vi "Access insert values.vi"(5 "是否创建唯一键":bool, 6 "Password":string, 7 "data":variant[](array[variant]), 8 "error in (no error)":errorcluster, 9 "columns外部输入":T1, 10 "database":string="database1.mdb", 11 "table":string) -> (0 "error out":errorcluster)   [LabVIEW 2016, in "Access Lib.lvlib"]
uses:
  Access Lib.lvlib
  <vilib>/addons/database/Auxilliary.llb/DB Tools Transaction.ctl
  <vilib>/addons/database/Auxilliary.llb/DB Tools Isolation Level.ctl
  <vilib>/addons/database/Auxilliary.llb/DB Tools Column Info.ctl
  <vilib>/addons/database/Auxilliary.llb/DB Tools DataTypes.ctl
  <vilib>/addons/database/Auxilliary.llb/DB Tools Parameter Info.ctl
  <vilib>/addons/database/Auxilliary.llb/DB Tools Parameter Dir.ctl
  <vilib>/addons/database/Connection.llb/DB Tools Open Connec (String).vi
  <vilib>/addons/database/Connection.llb/Conn Transaction.vi
  <vilib>/addons/database/Connection.llb/Conn Execute.vi
  <vilib>/addons/database/Recordset.llb/Rec Destroy - Connection.vi
  <vilib>/addons/database/Command.llb/Cmd Set Parameter Value (C).vi
  <vilib>/addons/database/Command.llb/Cmd Execute.vi
  <vilib>/addons/database/Recordset.llb/Rec Destroy - Command.vi
  <vilib>/addons/database/Command.llb/Cmd Delete.vi
  <vilib>/addons/database/NI_Database_API.lvlib
  <vilib>/Utility/VariantDataType/VariantType.lvlib
panel:
  out "SN":string
  out "布尔":bool
  out "曲线截距":sgl
  out "曲线斜率":sgl
  out "二次多项式系数":sgl
  out "X":sgl
  out "检测值":sgl
  out "测试模式":enum16{"水样测试", "零点核查", "跨度核查"}(ring)
  out "当前数据时间":timestamp
  out "当前测量模式":string
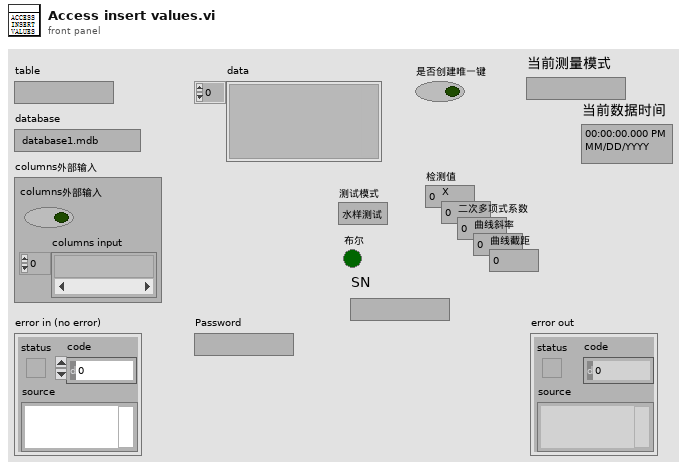
[diagram p1: front panel]
types:
  T1 = cluster{"columns外部输入":bool, "columns input":string[]}
  T2 = typedef "NI_Database_API.lvlib/DB Tools Isolation Level.ctl" = enum16{"chaos", "read uncommitted", "read committed", "repeatable read", "serializable"}
  T3 = typedef "NI_Database_API.lvlib/DB Tools Transaction.ctl" = enum16{"begin", "commit", "rollback"}
  T4 = typedef "NI_Database_API.lvlib/DB Tools Column Info.ctl" = cluster{"column name":string, "data type":T5, "size":i32, "allow null?":bool}
  T5 = typedef "NI_Database_API.lvlib/DB Tools DataTypes.ctl" = enum16{"String", "Long (I32)", "Single (SGL)", "Double (DBL)", "Date/Time", "Binary"}
  T6 = typedef "VariantType.lvlib/Type.ctl" = enum8{"Invalid Type", "Void", "I8", "I16", "I32", "I64", "U8", "U16", "U32", "U64", "Single Float", "Double Float", "Extended Float", "Single Complex", "Double Complex", "Extended Complex", "Enum U8", "Enum U16", "Enum U32", "Enum U64", "Single Float With Unit", "Double Float With Unit", "Extended Float With Unit", "Single Complex with Unit", "Double Complex with Unit", "Extended Complex with Unit", "Boolean", "String", "Path", "Picture", "Tag", "Array", "Cluster", "Variant", "LV Variant", "Waveform", "Timestamp", "Digital Waveform", "Digital Data", "ExpressData", "Refnum", "External Data", "VI", "Poly VI", "LabVIEW Class Instance", "Fixed Point"}
  T7 = typedef "NI_Database_API.lvlib/Conn ObjectReference.ctl" = refnum<k1>
  T8 = typedef "NI_Database_API.lvlib/DB Tools Parameter Info.ctl" = cluster{"parameter name":string, "type":T5, "direction":T9, "value":variant}
  T9 = typedef "NI_Database_API.lvlib/DB Tools Parameter Dir.ctl" = enum32{"Input", "Output", "Input/Output", "Return Value"}
  T10 = typedef "NI_Database_API.lvlib/Rec ObjectReference.ctl" = refnum<k1>
  T11 = typedef "LVDateTimeRec.ctl" = cluster{"秒数的小数部分":dbl, "秒":i32, "分":i32, "时":i32, "日":i32, "月":i32, "年":i32, "天数（周）":i32, "天数（年）":i32, "DST":i32}
  T12 = typedef "NI_Database_API.lvlib/Cmd ObjectReference.ctl" = refnum<k1>
  T13 = typedef "NI_Database_API.lvlib/Cmd-Rec Object Reference.ctl" = refnum<k1>
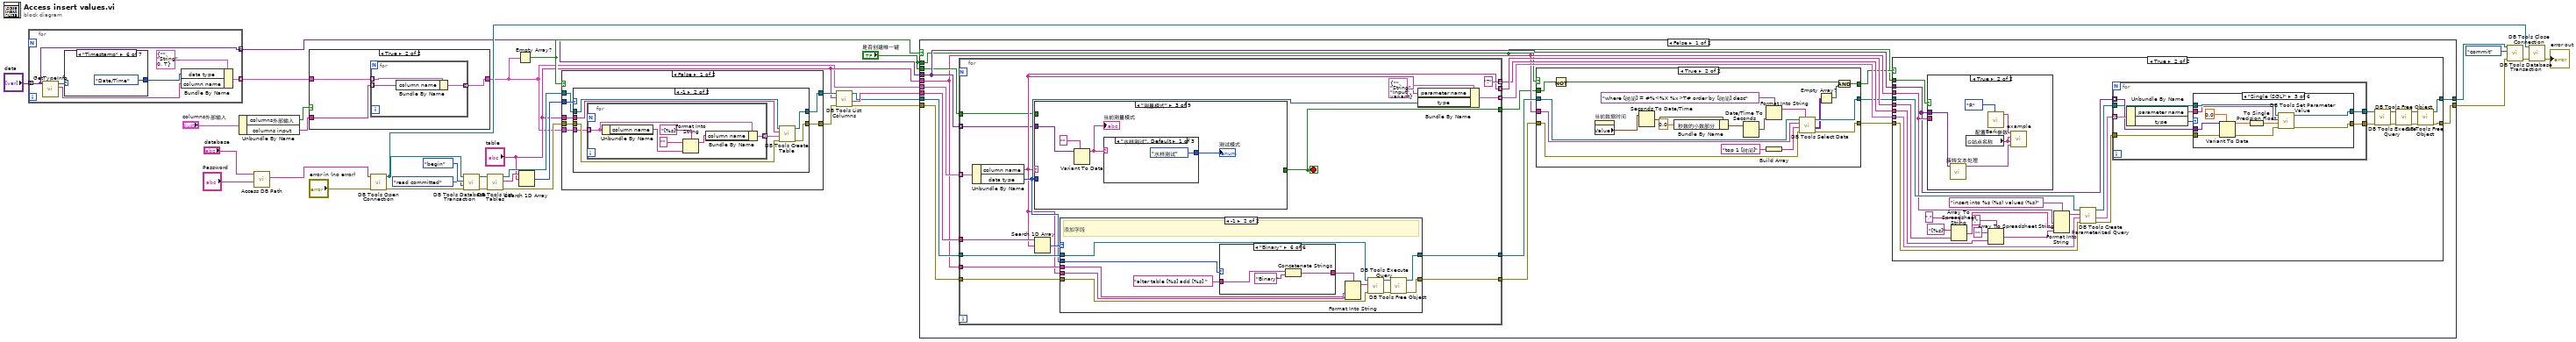
[diagram p0: block diagram]
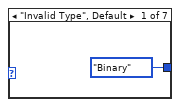
[diagram p3: hidden frame]
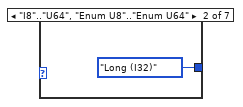
[diagram p4: hidden frame]
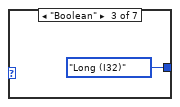
[diagram p5: hidden frame]
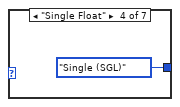
[diagram p6: hidden frame]
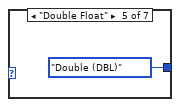
[diagram p7: hidden frame]
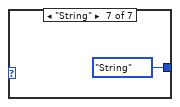
[diagram p8: hidden frame]
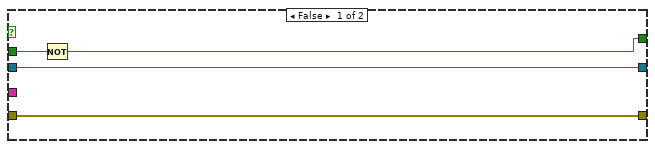
[diagram p11: hidden frame]
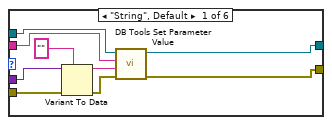
[diagram p14: hidden frame]
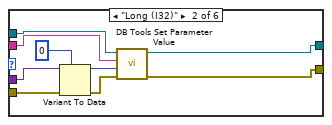
[diagram p15: hidden frame]
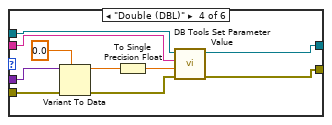
[diagram p16: hidden frame]
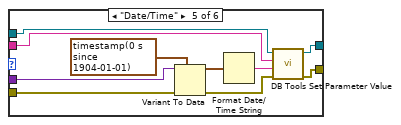
[diagram p17: hidden frame]
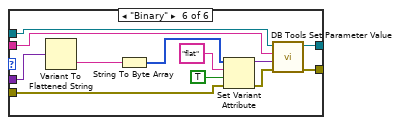
[diagram p18: hidden frame]
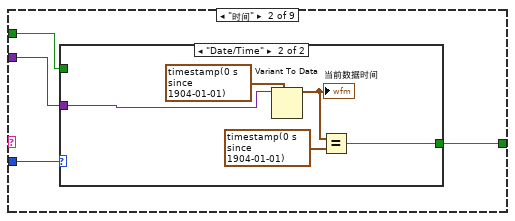
[diagram p20: hidden frame]
diagram:
  n1 = for {
    tunnel: [w35] -> w12 mode=indexing
    tunnel: [w37] -> w9 mode=indexing
    tunnel: "data" -> [w35] mode=indexing
    n2 = call <vilib>:"GetTypeInfo.vi"("Variant"=w35) -> ("Name"=w36:string, "Type Enum"=w39:T6)  [unwired: 6 in, 3 out]
    n3 = case shown="\"Timestamp\"" w39 {
      tunnel: [DB_Tools_DataTypes."Binary" ("data type") DB_Tools_DataTypes."Long (I32)" ("data type") DB_Tools_DataTypes."Long (I32)" ("data type") DB_Tools_DataTypes."Single (SGL)" ("data type") DB_Tools_DataTypes."Double (DBL)" ("data type") DB_Tools_DataTypes."Date/Time" ("data type") DB_Tools_DataTypes."String" ("data type")] -> w38
      frame "Invalid Type", Default {
      }
      frame "I8".."U64", "Enum U8".."Enum U64" {
      }
      frame "Boolean" {
      }
      frame "Single Float" {
      }
      frame "Double Float" {
      }
      frame "Timestamp" {
      }
      frame "String" {
      }
    }
    n4 = Bundle By Name(cluster=T4 {"column name"="", "data type"=enum."String", "size"=0, "allow null?"=TRUE} ("column information"), "data type"=w38, "column name"=w36) -> (w37:T4)
  }
  n5 = Unbundle By Name("columns外部输入") -> ("columns外部输入"=w7:bool, "columns input"=w8:string[])
  n6 = call "Access DB Path.vi"("Password"="Password", "database"="database") -> ("Connection information"=w5:string)  [unwired: 8 in, 1 out]
  n7 = case shown="True" w7 {
    tunnel: w9 -> [w48 w51]
    tunnel: [w48 w50] -> w6
    tunnel: w8 -> [_ w49]
    frame False {
    }
    frame True {
      n8 = for {
        tunnel: w51 -> [w54] mode=indexing
        tunnel: [w53] -> w50 mode=indexing
        tunnel: w49 -> [w52] mode=indexing
        n9 = Bundle By Name(cluster=w54, "column name"=w52) -> (w53:T4)
      }
    }
  }
  n10 = call-poly <vilib>:"DB Tools Open Connection.vi"("error in (no error)"="error in (no error)", "connection information"=w5) -> ("error out"=w19:errorcluster, "connection reference"=w16:T7)  [unwired: 6 in]
  n11 = call-poly <vilib>:"DB Tools Database Transaction.vi"("error in (no error)"=w19, "isolation level (chaos)"=DB_Tools_Isolation_Level."read committed", "operation (begin)"=DB_Tools_Transaction."begin", "connection reference"=w16) -> ("error out"=w18:errorcluster, "connection reference out"=w20:T7)  [unwired: 2 in]
  n12 = call <vilib>:"DB Tools List Tables.vi"("error in (no error)"=w18, "connection reference"=w20) -> ("error out"=w27:errorcluster, "tables"=w29:string[], "connection reference out"=w17:T7)  [unwired: 3 in]
  n13 = Empty Array?(array=w6) -> (empty?=w14:bool)
  n14 = Search 1D Array(1D array=w29, element="table") -> (index of element=w28:i32)  [unwired: 1 in]
  n15 = case shown="False" w14 {
    tunnel: w28 -> [w61 _]
    tunnel: w27 -> [w60 w77]
    tunnel: [w59 w78] -> w25
    tunnel: [w58 w77] -> w24
    tunnel: w17 -> [w57 w78]
    tunnel: "table" -> [w56 _]
    tunnel: w6 -> [w55 _]
    frame False {
      n16 = case shown="-1" w61 {
        tunnel: w57 -> [w63 w70]
        tunnel: w60 -> [w62 w69]
        tunnel: w56 -> [_ w68]
        tunnel: w55 -> [_ w65]
        tunnel: [w63 w67] -> w59
        tunnel: [w62 w66] -> w58
        frame 0, Default {
        }
        frame -1 {
          n17 = for {
            tunnel: w65 -> [w72] mode=indexing
            tunnel: [w71] -> w64 mode=indexing
            n18 = Unbundle By Name(w72) -> ("column name"=w76:string)
            n19 = Format Into String(format string="[%s]" ("格式字符串"), initial string="" ("初始字符串"), w76) -> (resulting string=w73:string)  [unwired: 1 in, 1 out]
            n20 = Bundle By Name(cluster=w72, "column name"=w73) -> (w71:T4)
          }
          n21 = call <vilib>:"DB Tools Create Table.vi"("error in (no error)"=w69, "column information"=w64, "table"=w68, "connection reference"=w70) -> ("error out"=w66:errorcluster, "connection reference out"=w67:T7)  [unwired: 4 in]
        }
      }
    }
    frame True {
    }
  }
  n22 = call <vilib>:"DB Tools List Columns.vi"("error in (no error)"=w24, "table"="table", "connection reference"=w25) -> ("error out"=w3:errorcluster, "columns"=w26:string[], "connection reference out"=w4:T7)  [unwired: 1 in, 1 out]
  n23 = case shown="False" w14 {
    tunnel: w26 -> [w97 _]
    tunnel: w3 -> [w96 w306]
    tunnel: [w92 w307] -> w22
    tunnel: [w91 w306] -> w21
    tunnel: w12 -> [w88 _]
    tunnel: w4 -> [w90 w307]
    tunnel: "table" -> [w82 _]
    tunnel: w6 -> [w89 _]
    tunnel: "是否创建唯一键" -> [w87 _]
    tunnel: "是否创建唯一键" -> [w79 _]
    frame False {
      n24 = for {
        tunnel: w90 -> [w236]
        tunnel: w97 -> [w238]
        tunnel: w96 -> [w235]
        tunnel: [w234] -> w84
        tunnel: w82 -> [w233]
        tunnel: w89 -> [w232] mode=indexing
        tunnel: [w230] -> w95 mode=indexing
        tunnel: [w226] -> w94 mode=indexing
        tunnel: ["?"] -> w93 mode=indexing
        tunnel: [w228] -> w86
        tunnel: w88 -> [w225] mode=indexing
        tunnel: [w224] -> w81
        tunnel: w87 -> [w223]
        stop <- w224 stop-if-true
        n25 = Unbundle By Name(w232) -> ("column name"=w226:string, "data type"=w227:T5)
        n26 = case shown="\"测量模式\"" w226 {
          tunnel: w227 -> [_ w242 _ _ _ _ _ _ _]
          tunnel: w225 -> [_ w241 w251 w257 w260 w263 w266 w269 w272]
          tunnel: [_ w240 _ _ _ _ _ _ _] -> w224
          tunnel: w223 -> [_ w239 _ _ _ _ _ _ _]
          frame "假", Default {
          }
          frame "时间" {
            n27 = case shown="\"Date/Time\"" w242 {
              tunnel: w241 -> [_ w247]
              tunnel: [_ w243] -> w240
              tunnel: w239 -> [_ _]
              frame "String", Default {
              }
              frame "Date/Time" {
                n28 = Variant To Data(type=timestamp(0 s since 1904-01-01) ("时间标识"), Variant=w247) -> (data=w245:timestamp)  [unwired: 1 in, 1 out]
                "当前数据时间" <- w245
                n29 = Equal?(x=w245, y=timestamp(0 s since 1904-01-01) ("时间标识")) -> (x = y?=w243:bool)
              }
            }
          }
          frame "测量模式" {
            n30 = Variant To Data(type="", Variant=w251) -> (data=w249:string)  [unwired: 1 in, 1 out]
            "当前测量模式" <- w249
            n31 = case shown="\"水样测试\", Default" w249 {
              tunnel: [enum16{"水样测试", "零点核查", "跨度核查"}."水样测试" ("测试模式") enum16{"水样测试", "零点核查", "跨度核查"}."零点核查" ("测试模式") enum16{"水样测试", "零点核查", "跨度核查"}."跨度核查" ("测试模式")] -> w248
              frame "水样测试", Default {
              }
              frame "零点核查" {
              }
              frame "跨度核查" {
              }
            }
            "测试模式" <- w248
          }
          frame "检测值" {
            n32 = Variant To Data(type=sgl 0.0, Variant=w257) -> (data=→"检测值":sgl)  [unwired: 1 in, 1 out]
            "布尔" <- TRUE ("布尔")
          }
          frame "X0" {
            n33 = Variant To Data(type=sgl 0.0, Variant=w260) -> (data=→"X":sgl)  [unwired: 1 in, 1 out]
          }
          frame "二次多项式系数" {
            n34 = Variant To Data(type=sgl 0.0, Variant=w263) -> (data=→"二次多项式系数":sgl)  [unwired: 1 in, 1 out]
          }
          frame "曲线斜率" {
            n35 = Variant To Data(type=sgl 0.0, Variant=w266) -> (data=→"曲线斜率":sgl)  [unwired: 1 in, 1 out]
          }
          frame "曲线截距" {
            n36 = Variant To Data(type=sgl 0.0, Variant=w269) -> (data=→"曲线截距":sgl)  [unwired: 1 in, 1 out]
          }
          frame "SN" {
            n37 = Variant To Data(type="", Variant=w272) -> (data=→"SN":string)  [unwired: 1 in, 1 out]
          }
        }
        n38 = Search 1D Array(1D array=w238, element=w226) -> (index of element=w237:i32)  [unwired: 1 in]
        n39 = case shown="-1" w237 {
          tunnel: [w275 w284] -> w234
          tunnel: w236 -> [w274 w283]
          tunnel: w226 -> [_ w282]
          tunnel: w235 -> [w275 w281]
          tunnel: w233 -> [_ w280]
          tunnel: w227 -> [_ w278]
          tunnel: [w274 w276] -> w228
          frame 0, Default {
          }
          frame -1 {
            # "添加字段"
            n40 = case shown="\"Binary\"" w278 {
              tunnel: "alter table [%s] add [%s] " -> [w290 w293 w296 w299 w302 w305]
              tunnel: [w289 w292 w295 w298 w301 w304] -> w277
              frame "String", Default {
                n41 = Concatenate Strings(w290, "String" ("字符串")) -> (w289:string)
              }
              frame "Long (I32)" {
                n42 = Concatenate Strings(w293, "Long" ("字符串")) -> (w292:string)
              }
              frame "Single (SGL)" {
                n43 = Concatenate Strings(w296, "Single" ("字符串")) -> (w295:string)
              }
              frame "Double (DBL)" {
                n44 = Concatenate Strings(w299, "Double" ("字符串")) -> (w298:string)
              }
              frame "Date/Time" {
                n45 = Concatenate Strings(w302, "TimeStamp" ("字符串")) -> (w301:string)
              }
              frame "Binary" {
                n46 = Concatenate Strings(w305, "Binary" ("字符串")) -> (w304:string)
              }
            }
            n47 = Format Into String(format string=w277, w280, w282) -> (resulting string=w285:string)  [unwired: 2 in, 1 out]
            n48 = call-poly <vilib>:"DB Tools Execute Query.vi"("error in (no error)"=w281, "SQL query"=w285, "connection reference"=w283) -> ("error out"=w286:errorcluster, "recordset reference"=w287:T10)  [unwired: 5 in]
            n49 = call-poly <vilib>:"DB Tools Free Object.vi"("error in (no error)"=w286, "recordset reference"=w287) -> ("error out"=w284:errorcluster, "connection reference"=w276:T7)  [unwired: 8 in]
          }
        }
        n50 = Bundle By Name(cluster=T8 {"parameter name"="", "type"=enum."String", "direction"=enum."Input", "value"=variant} ("parameter information"), "parameter name"=w226, "type"=w227) -> (w230:T8)
      }
      n51 = case shown="True" w79 {
        tunnel: w86 -> [w101 w118]
        tunnel: [w101 w117] -> w85
        tunnel: w84 -> [w100 w116]
        tunnel: [w100 w115] -> w83
        tunnel: w82 -> [_ w114]
        tunnel: w81 -> [w99 w103]
        tunnel: [w98 w105] -> w80
        frame False {
          n52 = Not(x=w99) -> (.not. x?=w98:bool)
        }
        frame True {
          n53 = Not(x=w103) -> (.not. x?=w102:bool)
          n54 = property on="当前数据时间" class="AbsTime (strict)"() -> ("Value"=w111:timestamp)  [unwired: 2 in, 2 out]
          n55 = Seconds To Date/Time(time stamp (now)=w111) -> (date time rec=w110:T11)  [unwired: 1 in]
          n56 = Bundle By Name(cluster=w110, "秒数的小数部分"=0.0) -> (w107:T11)
          n57 = Date/Time To Seconds(2:w107) -> (0:w108:timestamp)  [unwired: 1 in]
          n58 = Format Into String(format string="where [时间] = #%<%X %x>T# order by [时间] desc" ("condition"), w108) -> (resulting string=w113:string)  [unwired: 2 in, 1 out]
          n59 = Build Array("top 1 [时间]") -> (w120:string[])
          n60 = call <vilib>:"DB Tools Select Data.vi"("condition"=w113, "error in (no error)"=w116, "columns"=w120, "table"=w114, "connection reference"=w118) -> ("error out"=w115:errorcluster, "data"=w106:variant[][], "connection reference out"=w117:T7)  [unwired: 1 in]
          n61 = Empty Array?(array=w106) -> (empty?=w104:bool)
          n62 = And(x=w102, y=w104) -> (x .and. y?=w105:bool)
        }
      }
      n63 = case shown="True" w80 {
        tunnel: w95 -> [_ w149]
        tunnel: w94 -> [_ w143]
        tunnel: w93 -> [_ w141]
        tunnel: [w122 w131] -> w92
        tunnel: [w121 w130] -> w91
        tunnel: w85 -> [w122 w128]
        tunnel: w83 -> [w121 w126]
        tunnel: w82 -> [_ w125]
        tunnel: w88 -> [_ w124]
        tunnel: w79 -> [_ w123]
        frame False {
        }
        frame True {
          n64 = case shown="True" w123 {
            tunnel: w125 -> [_ _]
            tunnel: w124 -> [_ w154]
            frame False {
            }
            frame True {
              n65 = call "簇转文本处理.vi"("data"=w154) -> ("output"=w153:string)  [unwired: 10 in]
              n66 = global read "非断电保持全局变量.vi" "站点名称"() -> (w150:string)
              n67 = call "配置Bark参数.vi"("FUN"=enum16{"W", "R"}."R") -> ("URLs 2"=w151:string[])  [unwired: 10 in]
              n68 = call "example.vi"("Message"=w153, "Title"=w150, "Group"=w150, "urls"=w151) -> ()  [unwired: 8 in]
            }
          }
          n69 = Array To Spreadsheet String(delimiter (Tab)="," ("分隔符(Tab)"), array=w143, 3:"[%s]" ("格式字符串")) -> (spreadsheet string=w142:string)
          n70 = Array To Spreadsheet String(delimiter (Tab)="," ("分隔符(Tab)"), array=w141, 3:"" ("格式字符串")) -> (spreadsheet string=w140:string)
          n71 = Format Into String(format string="insert into %s (%s) values (%s)" ("格式字符串"), w125, w142, w140) -> (resulting string=w139:string)  [unwired: 2 in, 1 out]
          n72 = call <vilib>:"DB Tools Create Parameterized Query.vi"("error in (no error)"=w126, "parameters"=w149, "SQL query"=w139, "connection reference"=w128) -> ("error out"=w138:errorcluster, "parameters out"=w137:T8[], "command reference"=w129:T12)  [unwired: 3 in]
          n73 = for {
            tunnel: w129 -> [w159]
            tunnel: w138 -> [w157]
            tunnel: w137 -> [w162] mode=indexing
            tunnel: w124 -> [w160] mode=indexing
            tunnel: [w156] -> w127
            tunnel: [w155] -> w136
            n74 = Unbundle By Name(w162) -> ("parameter name"=w158:string, "type"=w161:T5)
            n75 = case shown="\"Single (SGL)\"" w161 {
              tunnel: w160 -> [w166 w174 w184 w194 w210 w214]
              tunnel: w159 -> [w169 w178 w187 w198 w208 w222]
              tunnel: w158 -> [w168 w177 w183 w193 w203 w221]
              tunnel: w157 -> [w163 w172 w185 w195 w206 w213]
              tunnel: [w165 w176 w188 w197 w205 w220] -> w156
              tunnel: [w164 w175 w186 w196 w204 w219] -> w155
              frame "String", Default {
                n76 = Variant To Data(error in=w163, type="", Variant=w166) -> (data=w167:string, error out=w171:errorcluster)
                n77 = call-poly <vilib>:"DB Tools Set Parameter Value.vi"("error in (no error)"=w171, "value"=w167, "parameter index"=w168, "command reference"=w169) -> ("error out"=w164:errorcluster, "command reference out"=w165:T12)  [unwired: 4 in]
              }
              frame "Long (I32)" {
                n78 = Variant To Data(error in=w172, type=0, Variant=w174) -> (data=w179:i32, error out=w180:errorcluster)
                n79 = call-poly <vilib>:"DB Tools Set Parameter Value.vi"("error in (no error)"=w180, "value"=w179, "parameter index"=w177, "command reference"=w178) -> ("error out"=w175:errorcluster, "command reference out"=w176:T12)  [unwired: 4 in]
              }
              frame "Single (SGL)" {
                n80 = Variant To Data(error in=w185, type=sgl 0.0, Variant=w184) -> (data=w182:sgl, error out=w190:errorcluster)
                n81 = To Single Precision Float(number=w182) -> (single precision float=w181:sgl)
                n82 = call-poly <vilib>:"DB Tools Set Parameter Value.vi"("error in (no error)"=w190, "value"=w181, "parameter index"=w183, "command reference"=w187) -> ("error out"=w186:errorcluster, "command reference out"=w188:T12)  [unwired: 4 in]
              }
              frame "Double (DBL)" {
                n83 = Variant To Data(error in=w195, type=0.0, Variant=w194) -> (data=w192:dbl, error out=w200:errorcluster)
                n84 = To Single Precision Float(number=w192) -> (single precision float=w191:sgl)
                n85 = call-poly <vilib>:"DB Tools Set Parameter Value.vi"("error in (no error)"=w200, "value"=w191, "parameter index"=w193, "command reference"=w198) -> ("error out"=w196:errorcluster, "command reference out"=w197:T12)  [unwired: 4 in]
              }
              frame "Date/Time" {
                n86 = Variant To Data(error in=w206, type=timestamp(0 s since 1904-01-01) ("时间标识"), Variant=w210) -> (data=w202:timestamp, error out=w207:errorcluster)
                n87 = Format Date/Time String(seconds (now)=w202) -> (date/time string=w201:string)  [unwired: 2 in]
                n88 = call-poly <vilib>:"DB Tools Set Parameter Value.vi"("error in (no error)"=w207, "value"=w201, "parameter index"=w203, "command reference"=w208) -> ("error out"=w204:errorcluster, "command reference out"=w205:T12)  [unwired: 4 in]
              }
              frame "Binary" {
                n89 = Variant To Flattened String(Variant=w214) -> (data string=w215:string)  [unwired: 1 out]
                n90 = String To Byte Array(string=w215) -> (unsigned byte array=w218:u8[])
                n91 = Set Variant Attribute(Variant=w218, name="flat", value=TRUE, error in=w213) -> (Variant out=w211:variant, error out=w212:errorcluster)  [unwired: 1 out]
                n92 = call-poly <vilib>:"DB Tools Set Parameter Value.vi"("error in (no error)"=w212, "value"=w211, "parameter index"=w221, "command reference"=w222) -> ("error out"=w219:errorcluster, "command reference out"=w220:T12)  [unwired: 4 in]
              }
            }
          }
          n93 = call-poly <vilib>:"DB Tools Execute Query.vi"("error in (no error)"=w136, "command reference"=w127) -> ("error out"=w134:errorcluster, "command-recordset reference"=w135:T13)  [unwired: 6 in]
          n94 = call-poly <vilib>:"DB Tools Free Object.vi"("error in (no error)"=w134, "command-recordset reference"=w135) -> ("error out"=w132:errorcluster, "command reference"=w133:T12)  [unwired: 8 in]
          n95 = call-poly <vilib>:"DB Tools Free Object.vi"("error in (no error)"=w132, "command reference"=w133) -> ("error out"=w130:errorcluster, "connection reference"=w131:T7)  [unwired: 8 in]
        }
      }
    }
    frame True {
    }
  }
  n96 = call-poly <vilib>:"DB Tools Database Transaction.vi"("error in (no error)"=w21, "operation (begin)"=DB_Tools_Transaction."commit", "connection reference"=w22) -> ("error out"=w23:errorcluster)  [unwired: 3 in, 1 out]
  n97 = call <vilib>:"DB Tools Close Connection.vi"("error in (no error)"=w23, "connection reference"=w16) -> ("error out"=→"error out":errorcluster)  [unwired: 5 in]
